vi "Condition checker.vi"(0 "Condition name":string, 2 "Condition comparator":string, 3 "Condition value":dbl) -> (7 "Condition in spec?":bool)   [LabVIEW 2014]
uses:
  Controls/ConditionsGlobal.vi
  Controls/ResultsGlobal.vi
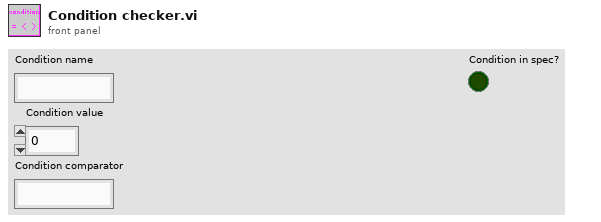
[diagram p1: front panel]
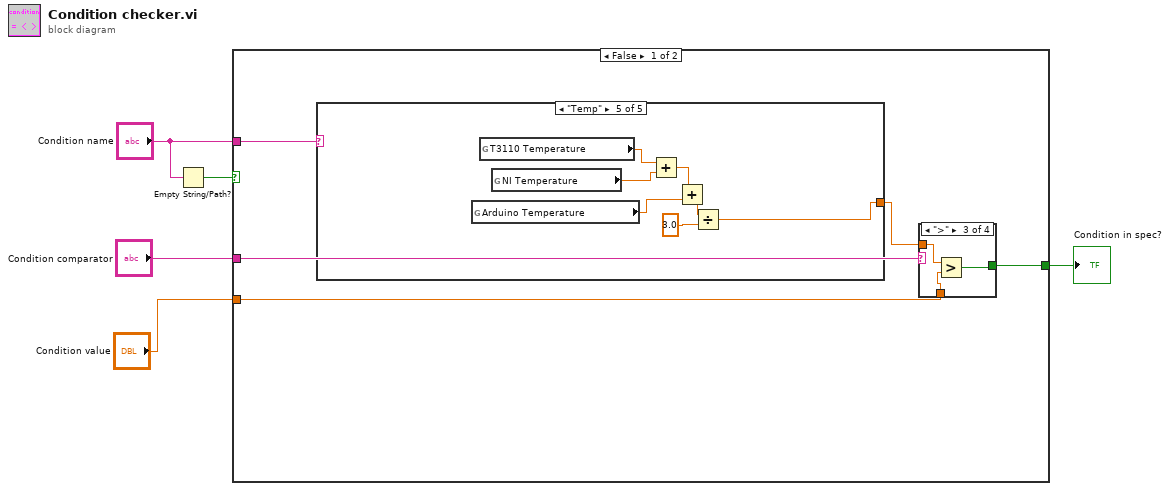
[diagram p0: block diagram]
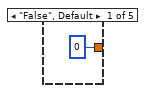
[diagram p2: hidden frame]
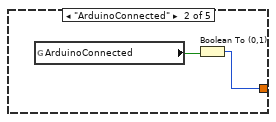
[diagram p3: hidden frame]
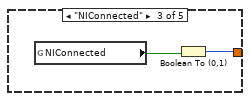
[diagram p4: hidden frame]
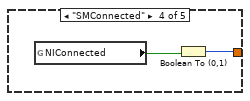
[diagram p5: hidden frame]
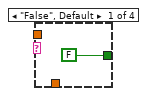
[diagram p6: hidden frame]
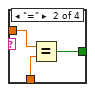
[diagram p7: hidden frame]
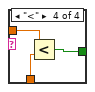
[diagram p8: hidden frame]
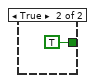
[diagram p9: hidden frame]
diagram:
  n1 = Empty String/Path?(string/path="Condition name") -> (empty?=w1:bool)
  n2 = case shown="False" w1 {
    tunnel: "Condition value" -> [w9 _]
    tunnel: "Condition comparator" -> [w8 _]
    tunnel: [w7 TRUE] -> w3
    tunnel: "Condition name" -> [w6 _]
    frame False {
      n3 = case shown="\"Temp\"" w6 {
        tunnel: [0 w12 w14 w16 w18] -> w10
        frame "False", Default {
        }
        frame "ArduinoConnected" {
          n4 = global read "ConditionsGlobal.vi" "ArduinoConnected"() -> (w13:bool)
          n5 = Boolean To (0,1)(Boolean=w13) -> (0, 1=w12:i16)
        }
        frame "NIConnected" {
          n6 = global read "ConditionsGlobal.vi" "NIConnected"() -> (w15:bool)
          n7 = Boolean To (0,1)(Boolean=w15) -> (0, 1=w14:i16)
        }
        frame "SMConnected" {
          n8 = global read "ConditionsGlobal.vi" "NIConnected"() -> (w17:bool)
          n9 = Boolean To (0,1)(Boolean=w17) -> (0, 1=w16:i16)
        }
        frame "Temp" {
          n10 = global read "ResultsGlobal.vi" "Arduino Temperature"() -> (w21:dbl)
          n11 = global read "ResultsGlobal.vi" "T3110 Temperature"() -> (w19:dbl)
          n12 = global read "ResultsGlobal.vi" "NI Temperature"() -> (w20:dbl)
          n13 = Add(x=w19, y=w20) -> (x+y=w22:dbl)
          n14 = Add(x=w22, y=w21) -> (x+y=w23:dbl)
          n15 = Divide(x=w23, y=3.0) -> (x/y=w18:dbl)
        }
      }
      n16 = case shown="\">\"" w8 {
        tunnel: w10 -> [_ w28 w31 w34]
        tunnel: w9 -> [_ w27 w29 w33]
        tunnel: [FALSE w26 w30 w32] -> w7
        frame "False", Default {
        }
        frame "=" {
          n17 = Equal?(x=w28, y=w27) -> (x = y?=w26:bool)
        }
        frame ">" {
          n18 = Greater?(x=w31, y=w29) -> (0:w30:bool)
        }
        frame "<" {
          n19 = Less?(x=w34, y=w33) -> (x < y?=w32:bool)
        }
      }
    }
    frame True {
    }
  }
  "Condition in spec?" <- w3
